vi "Angle fixed overlay.vi"(9 "Fixed FOV parameters":T2, 10 "Mouse release point":cluster{"X":sgl, "Y":sgl}, 11 "Angle":T1) -> (1 "Overlay Coordinates":cluster{"X":sgl, "Y":sgl}[](array[cluster]), 2 "Mouse release point out":cluster{"X":sgl, "Y":sgl}, 3 "Angle parameters out":T1)   [LabVIEW 2019]
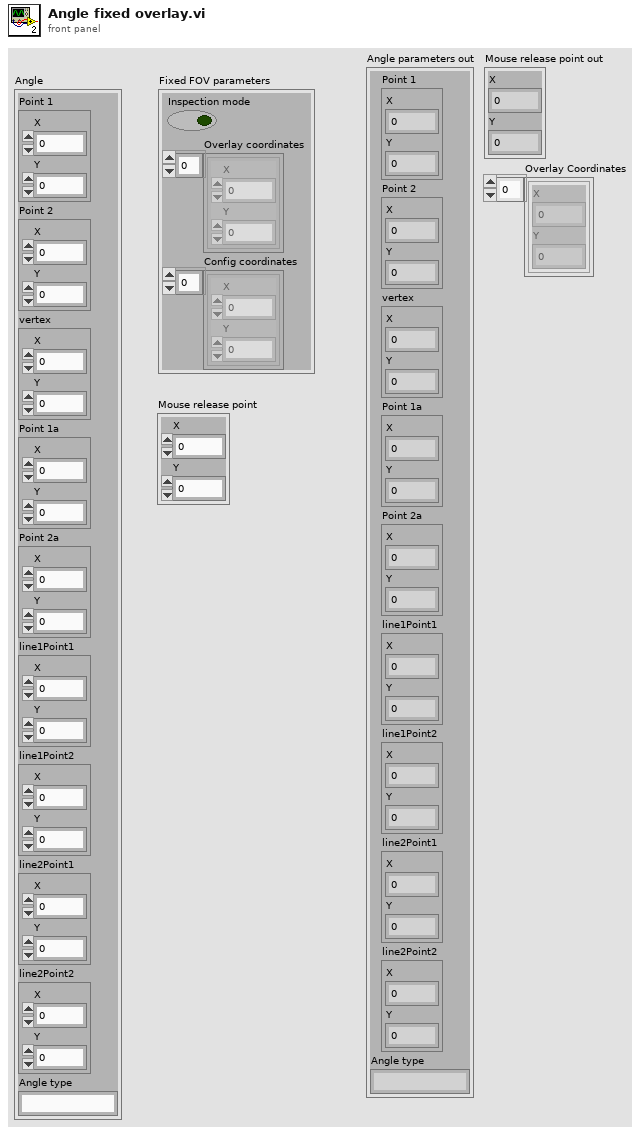
[diagram p1: front panel]
types:
  T1 = cluster{"Point 1":cluster{"X":sgl, "Y":sgl}, "Point 2":cluster{"X":sgl, "Y":sgl}, "vertex":cluster{"X":sgl, "Y":sgl}, "Point 1a":cluster{"X":sgl, "Y":sgl}, "Point 2a":cluster{"X":sgl, "Y":sgl}, "line1Point1":cluster{"X":sgl, "Y":sgl}, "line1Point2":cluster{"X":sgl, "Y":sgl}, "line2Point1":cluster{"X":sgl, "Y":sgl}, "line2Point2":cluster{"X":sgl, "Y":sgl}, "Angle type":string}
  T2 = cluster{"Inspection mode":bool, "Overlay coordinates":cluster{"X":sgl, "Y":sgl}[], "Config coordinates":cluster{"X":sgl, "Y":sgl}[]}
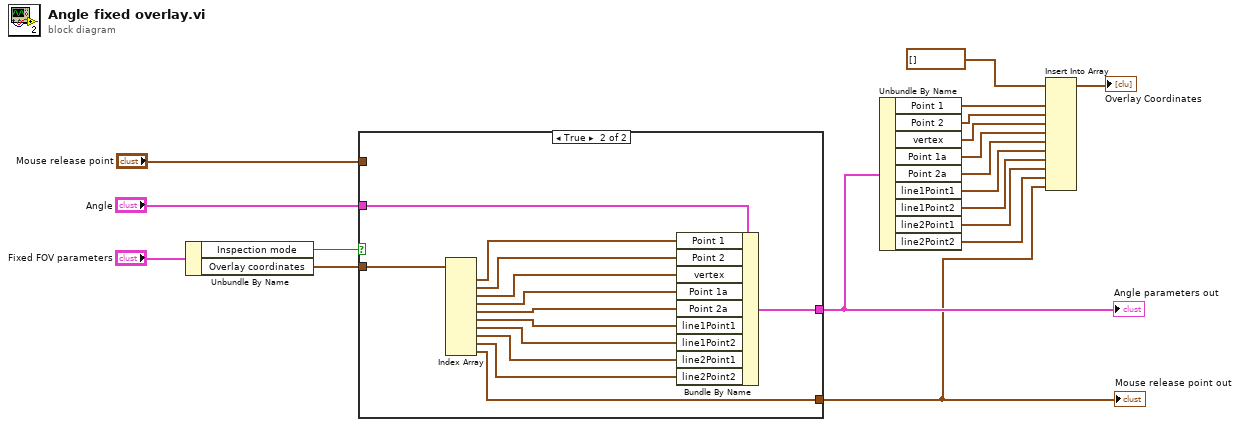
[diagram p0: block diagram]
diagram:
  n1 = Unbundle By Name("Fixed FOV parameters") -> ("Inspection mode"=w17:bool, "Overlay coordinates"=w16:cluster{"X":sgl, "Y":sgl}[])
  n2 = case shown="True" w17 {
    tunnel: w16 -> [_ w33]
    tunnel: "Mouse release point" -> [w19 _]
    tunnel: "Angle" -> [w20 w32]
    tunnel: [w19 w22] -> w2
    tunnel: [w20 w21] -> w13
    frame False {
    }
    frame True {
      n3 = Index Array(array=w33) -> (element #1=w31:cluster{"X":sgl, "Y":sgl}, element #2=w30:cluster{"X":sgl, "Y":sgl}, element #3=w29:cluster{"X":sgl, "Y":sgl}, element #4=w28:cluster{"X":sgl, "Y":sgl}, element #5=w27:cluster{"X":sgl, "Y":sgl}, element #6=w26:cluster{"X":sgl, "Y":sgl}, element #7=w25:cluster{"X":sgl, "Y":sgl}, element #8=w24:cluster{"X":sgl, "Y":sgl}, element #9=w23:cluster{"X":sgl, "Y":sgl}, element #10=w22:cluster{"X":sgl, "Y":sgl})  [unwired: 10 in]
      n4 = Bundle By Name(cluster=w32, "Point 1"=w31, "Point 2"=w30, "vertex"=w29, "Point 1a"=w28, "Point 2a"=w27, "line1Point1"=w26, "line1Point2"=w25, "line2Point1"=w24, "line2Point2"=w23) -> (w21:T1)
    }
  }
  "Angle parameters out" <- w13
  "Mouse release point out" <- w2
  n5 = Unbundle By Name(w13) -> ("Point 1"=w12:cluster{"X":sgl, "Y":sgl}, "Point 2"=w10:cluster{"X":sgl, "Y":sgl}, "vertex"=w9:cluster{"X":sgl, "Y":sgl}, "Point 1a"=w8:cluster{"X":sgl, "Y":sgl}, "Point 2a"=w7:cluster{"X":sgl, "Y":sgl}, "line1Point1"=w6:cluster{"X":sgl, "Y":sgl}, "line1Point2"=w5:cluster{"X":sgl, "Y":sgl}, "line2Point1"=w4:cluster{"X":sgl, "Y":sgl}, "line2Point2"=w3:cluster{"X":sgl, "Y":sgl})
  n6 = Insert Into Array(array=cluster{"X":sgl, "Y":sgl}[] [], new element #1=w12, new element #2=w10, new element #3=w9, new element #4=w8, new element #5=w7, new element #6=w6, new element #7=w5, new element #8=w4, new element #9=w3, new element #10=w2) -> (→"Overlay Coordinates":cluster{"X":sgl, "Y":sgl}[])  [unwired: 1 in]
